vi "Coordinate MinMax.vi"(11 "Coordinates":i32[][](array[numeric])) -> (1 "Min Coordinate Value":i32, 3 "Max Coordinate Value":i32)   [LabVIEW 2019]
doc: "Find the min and max values of all coordinates provided."
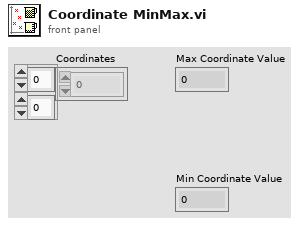
[diagram p1: front panel]
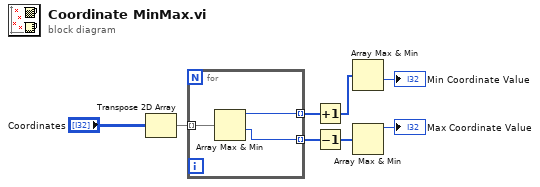
[diagram p0: block diagram]
diagram:
  n1 = Transpose 2D Array(2D array="Coordinates") -> (transposed array=w1:i32[][])
  n2 = for {
    tunnel: w1 -> [w11] mode=indexing
    tunnel: [w10] -> w3 mode=indexing
    tunnel: [w9] -> w2 mode=indexing
    n3 = Array Max & Min(array=w11) -> (max value=w10:i32, min value=w9:i32)  [unwired: 2 out]
  }
  n4 = Increment(x=w3) -> (x+1=w4:i32[])
  n5 = Decrement(x=w2) -> (x-1=w5:i32[])
  n6 = Array Max & Min(array=w4) -> (min value=→"Min Coordinate Value":i32)  [unwired: 3 out]
  n7 = Array Max & Min(array=w5) -> (max value=→"Max Coordinate Value":i32)  [unwired: 3 out]
